vi "Configure Channel Order & Numbers By Wiring.vi"(11 "wiring":T3) -> (1 "simulated signal definitions":T1(array[cluster]), 2 "number of channels":u8, 3 "AI data channel order":T2[](array[typedef]), 4 "voltage#":i32, 6 "current#":i32)   [LabVIEW 2013]
uses:
  <vilib>/addons/Electrical Power/PQ/Common/Controls/ep_Wiring.ctl
  <vilib>/addons/Electrical Power/PQ/Common/Controls/ep_AI Data Channel.ctl
  <vilib>/addons/Electrical Power/PQ/NI_EP_Power Quality.lvlib
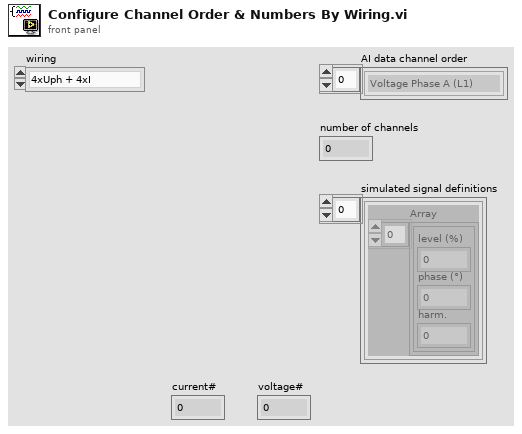
[diagram p1: front panel]
types:
  T1 = cluster{"Array":cluster{"level (%)":dbl, "phase (°)":dbl, "harm.":dbl}[]}[]
  T2 = typedef "NI_EP_Power Quality.lvlib/ep_AI Data Channel.ctl" = enum16{"Voltage Phase A (L1)", "Voltage Phase B (L2)", "Voltage Phase C (L3)", "Voltage Phase N (Neutral)", "Current Phase A (L1)", "Current Phase B (L2)", "Current Phase C (L3)", "Current Phase N (Neutral)"}
  T3 = typedef "NI_EP_Power Quality.lvlib/ep_Wiring.ctl" = enum16{"4xUph + 4xI", "3xUph + 4xI", "3xUline + 4xI", "3xUph + 3xI", "3xUline + 3xI", "3xUph + 2xI", "3xUline + 2xI", "1xUph + 1xI"}
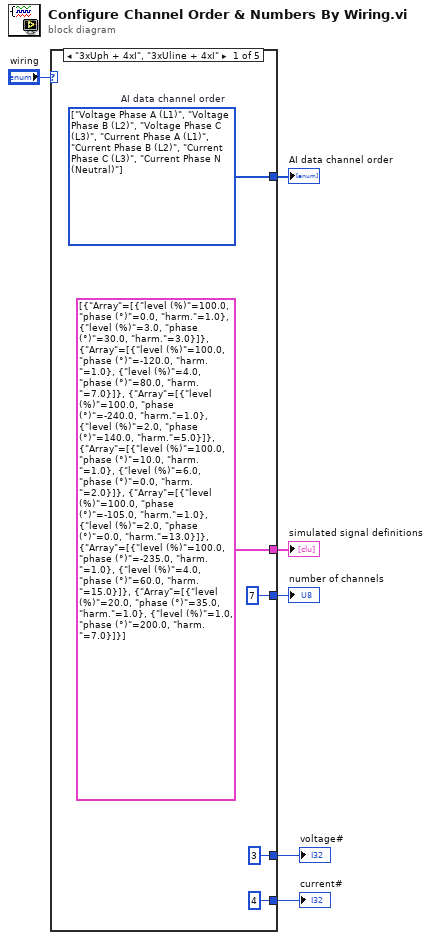
[diagram p0: block diagram]
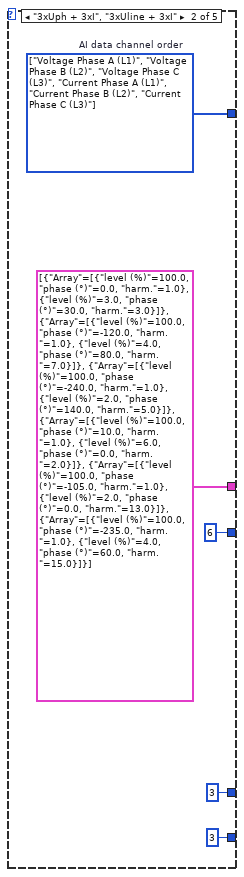
[diagram p2: hidden frame]
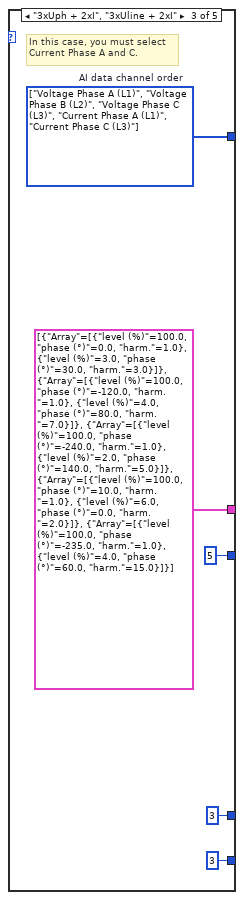
[diagram p3: hidden frame]
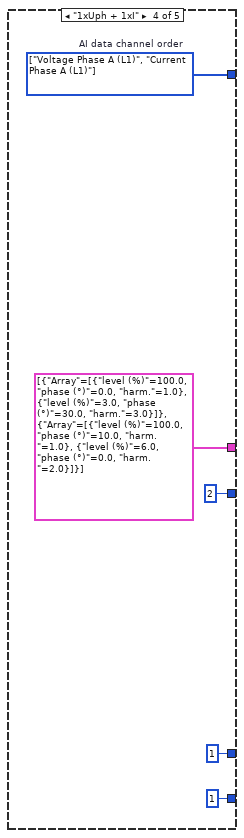
[diagram p4: hidden frame]
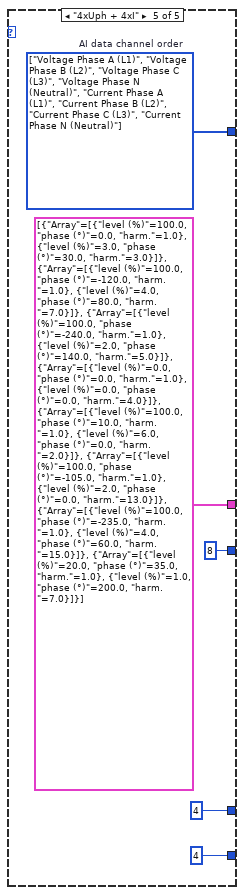
[diagram p5: hidden frame]
diagram:
  n1 = case shown="\"3xUph + 4xI\", \"3xUline + 4xI\"" "wiring" {
    tunnel: [w11 w16 w21 w26 w31] -> w5
    tunnel: [u8 7 ("number of channels") u8 6 ("number of channels") u8 5 ("number of channels") u8 2 ("number of channels") u8 8 ("number of channels")] -> w4
    tunnel: [T1 [{"Array"=[{"level (%)"=100.0, "phase (°)"=0.0, "harm."=1.0}, {"level (%)"=3.0, "phase (°)"=30.0, "harm."=3.0}]}, {"Array"=[{"level (%)"=100.0, "phase (°)"=-120.0, "harm."=1.0}, {"level (%)"=4.0, "phase (°)"=80.0, "harm."=7.0}]}, {"Array"=[{"level (%)"=100.0, "phase (°)"=-240.0, "harm."=1.0}, {"level (%)"=2.0, "phase (°)"=140.0, "harm."=5.0}]}, {"Array"=[{"level (%)"=100.0, "phase (°)"=10.0, "harm."=1.0}, {"level (%)"=6.0, "phase (°)"=0.0, "harm."=2.0}]}, {"Array"=[{"level (%)"=100.0, "phase (°)"=-105.0, "harm."=1.0}, {"level (%)"=2.0, "phase (°)"=0.0, "harm."=13.0}]}, {"Array"=[{"level (%)"=100.0, "phase (°)"=-235.0, "harm."=1.0}, {"level (%)"=4.0, "phase (°)"=60.0, "harm."=15.0}]}, {"Array"=[{"level (%)"=20.0, "phase (°)"=35.0, "harm."=1.0}, {"level (%)"=1.0, "phase (°)"=200.0, "harm."=7.0}]}] ("signal definition") T1 [{"Array"=[{"level (%)"=100.0, "phase (°)"=0.0, "harm."=1.0}, {"level (%)"=3.0, "phase (°)"=30.0, "harm."=3.0}]}, {"Array"=[{"level (%)"=100.0, "phase (°)"=-120.0, "harm."=1.0}, {"level (%)"=4.0, "phase (°)"=80.0, "harm."=7.0}]}, {"Array"=[{"level (%)"=100.0, "phase (°)"=-240.0, "harm."=1.0}, {"level (%)"=2.0, "phase (°)"=140.0, "harm."=5.0}]}, {"Array"=[{"level (%)"=100.0, "phase (°)"=10.0, "harm."=1.0}, {"level (%)"=6.0, "phase (°)"=0.0, "harm."=2.0}]}, {"Array"=[{"level (%)"=100.0, "phase (°)"=-105.0, "harm."=1.0}, {"level (%)"=2.0, "phase (°)"=0.0, "harm."=13.0}]}, {"Array"=[{"level (%)"=100.0, "phase (°)"=-235.0, "harm."=1.0}, {"level (%)"=4.0, "phase (°)"=60.0, "harm."=15.0}]}] ("signal definition") T1 [{"Array"=[{"level (%)"=100.0, "phase (°)"=0.0, "harm."=1.0}, {"level (%)"=3.0, "phase (°)"=30.0, "harm."=3.0}]}, {"Array"=[{"level (%)"=100.0, "phase (°)"=-120.0, "harm."=1.0}, {"level (%)"=4.0, "phase (°)"=80.0, "harm."=7.0}]}, {"Array"=[{"level (%)"=100.0, "phase (°)"=-240.0, "harm."=1.0}, {"level (%)"=2.0, "phase (°)"=140.0, "harm."=5.0}]}, {"Array"=[{"level (%)"=100.0, "phase (°)"=10.0, "harm."=1.0}, {"level (%)"=6.0, "phase (°)"=0.0, "harm."=2.0}]}, {"Array"=[{"level (%)"=100.0, "phase (°)"=-235.0, "harm."=1.0}, {"level (%)"=4.0, "phase (°)"=60.0, "harm."=15.0}]}] ("signal definition") T1 [{"Array"=[{"level (%)"=100.0, "phase (°)"=0.0, "harm."=1.0}, {"level (%)"=3.0, "phase (°)"=30.0, "harm."=3.0}]}, {"Array"=[{"level (%)"=100.0, "phase (°)"=10.0, "harm."=1.0}, {"level (%)"=6.0, "phase (°)"=0.0, "harm."=2.0}]}] ("signal definition") T1 [{"Array"=[{"level (%)"=100.0, "phase (°)"=0.0, "harm."=1.0}, {"level (%)"=3.0, "phase (°)"=30.0, "harm."=3.0}]}, {"Array"=[{"level (%)"=100.0, "phase (°)"=-120.0, "harm."=1.0}, {"level (%)"=4.0, "phase (°)"=80.0, "harm."=7.0}]}, {"Array"=[{"level (%)"=100.0, "phase (°)"=-240.0, "harm."=1.0}, {"level (%)"=2.0, "phase (°)"=140.0, "harm."=5.0}]}, {"Array"=[{"level (%)"=0.0, "phase (°)"=0.0, "harm."=1.0}, {"level (%)"=0.0, "phase (°)"=0.0, "harm."=4.0}]}, {"Array"=[{"level (%)"=100.0, "phase (°)"=10.0, "harm."=1.0}, {"level (%)"=6.0, "phase (°)"=0.0, "harm."=2.0}]}, {"Array"=[{"level (%)"=100.0, "phase (°)"=-105.0, "harm."=1.0}, {"level (%)"=2.0, "phase (°)"=0.0, "harm."=13.0}]}, {"Array"=[{"level (%)"=100.0, "phase (°)"=-235.0, "harm."=1.0}, {"level (%)"=4.0, "phase (°)"=60.0, "harm."=15.0}]}, {"Array"=[{"level (%)"=20.0, "phase (°)"=35.0, "harm."=1.0}, {"level (%)"=1.0, "phase (°)"=200.0, "harm."=7.0}]}] ("signal definition")] -> w3
    tunnel: [3 3 3 1 4] -> w2
    tunnel: [4 3 3 1 4] -> w1
    frame "3xUph + 4xI", "3xUline + 4xI" {
      w11 = T2[] [enum."Voltage Phase A (L1)", enum."Voltage Phase B (L2)", enum."Voltage Phase C (L3)", enum."Current Phase A (L1)", enum."Current Phase B (L2)", enum."Current Phase C (L3)", enum."Current Phase N (Neutral)"] items=["Voltage Phase A (L1)", "Voltage Phase B (L2)", "Voltage Phase C (L3)", "Voltage Phase N (Neutral)", "Current Phase A (L1)", "Current Phase B (L2)", "Current Phase C (L3)", "Current Phase N (Neutral)"]  # AI data channel order
    }
    frame "3xUph + 3xI", "3xUline + 3xI" {
      w16 = T2[] [enum."Voltage Phase A (L1)", enum."Voltage Phase B (L2)", enum."Voltage Phase C (L3)", enum."Current Phase A (L1)", enum."Current Phase B (L2)", enum."Current Phase C (L3)"] items=["Voltage Phase A (L1)", "Voltage Phase B (L2)", "Voltage Phase C (L3)", "Voltage Phase N (Neutral)", "Current Phase A (L1)", "Current Phase B (L2)", "Current Phase C (L3)", "Current Phase N (Neutral)"]  # AI data channel order
    }
    frame "3xUph + 2xI", "3xUline + 2xI" {
      w21 = T2[] [enum."Voltage Phase A (L1)", enum."Voltage Phase B (L2)", enum."Voltage Phase C (L3)", enum."Current Phase A (L1)", enum."Current Phase C (L3)"] items=["Voltage Phase A (L1)", "Voltage Phase B (L2)", "Voltage Phase C (L3)", "Voltage Phase N (Neutral)", "Current Phase A (L1)", "Current Phase B (L2)", "Current Phase C (L3)", "Current Phase N (Neutral)"]  # AI data channel order
      # "In this case, you must select Current Phase A and C."
    }
    frame "1xUph + 1xI" {
      w26 = T2[] [enum."Voltage Phase A (L1)", enum."Current Phase A (L1)"] items=["Voltage Phase A (L1)", "Voltage Phase B (L2)", "Voltage Phase C (L3)", "Voltage Phase N (Neutral)", "Current Phase A (L1)", "Current Phase B (L2)", "Current Phase C (L3)", "Current Phase N (Neutral)"]  # AI data channel order
    }
    frame "4xUph + 4xI" {
      w31 = T2[] [enum."Voltage Phase A (L1)", enum."Voltage Phase B (L2)", enum."Voltage Phase C (L3)", enum."Voltage Phase N (Neutral)", enum."Current Phase A (L1)", enum."Current Phase B (L2)", enum."Current Phase C (L3)", enum."Current Phase N (Neutral)"] items=["Voltage Phase A (L1)", "Voltage Phase B (L2)", "Voltage Phase C (L3)", "Voltage Phase N (Neutral)", "Current Phase A (L1)", "Current Phase B (L2)", "Current Phase C (L3)", "Current Phase N (Neutral)"]  # AI data channel order
    }
  }
  "AI data channel order" <- w5
  "number of channels" <- w4
  "simulated signal definitions" <- w3
  "voltage#" <- w2
  "current#" <- w1
